vi "Read SVW.vi"(11 "GUI in":refnum<class "GUI.lvclass">) -> (2 "SharedVariableWrapper.lvclass":refnum<class "SharedVariableWrapper.lvclass">)   [LabVIEW 2019, in "GUI.lvclass"]
uses:
  GUI.lvclass
  SV_Wrap/SharedVariableWrapper.lvclass
  GUI.lvclass/GUI.ctl
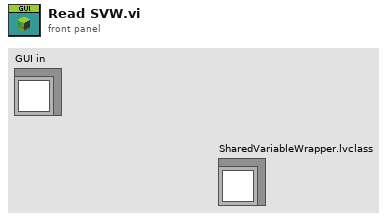
[diagram p1: front panel]
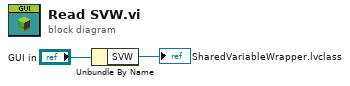
[diagram p0: block diagram]
diagram:
  n1 = Unbundle By Name("GUI in") -> ("SVW"=→"SharedVariableWrapper.lvclass":refnum<class "SharedVariableWrapper.lvclass">)
